vi "9_sub_Ntails.vi"(11 "Array":cluster{"PosX":i32, "PosY":i32}[](array[cluster])=[{"PosX"=0, "PosY"=0}, {"PosX"=0, "PosY"=1}, {"PosX"=0, "PosY"=2}, {"PosX"=0, "PosY"=3}, {"PosX"=0, "PosY"=3}, {"PosX"=1, "PosY"=4}, {"PosX"=2, "PosY"=4}, {"PosX"=3, "PosY"=4}, {"PosX"=3, "PosY"=4}, {"PosX"=4, "PosY"=3}, {"PosX"=4, "PosY"=2}, {"PosX"=4, "PosY"=2}, {"PosX"=4, "PosY"=2}, {"PosX"=4, "PosY"=2}, {"PosX"=3, "PosY"=3}, {"PosX"=3, "PosY"=4}, {"PosX"=3, "PosY"=4}, {"PosX"=3, "PosY"=4}, {"PosX"=3, "PosY"=4}, {"PosX"=2, "PosY"=3}, {"PosX"=2, "PosY"=2}, {"PosX"=2, "PosY"=1}, {"PosX"=2, "PosY"=1}, {"PosX"=2, "PosY"=1}]) -> (3 "Array 2":cluster{"PosX":i32, "PosY":i32}[](array[cluster]))   [LabVIEW 2021, in "2022.lvlib"]
uses:
  2022.lvlib
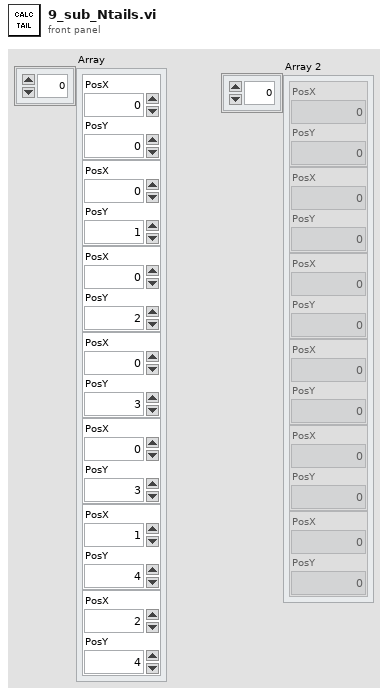
[diagram p1: front panel]
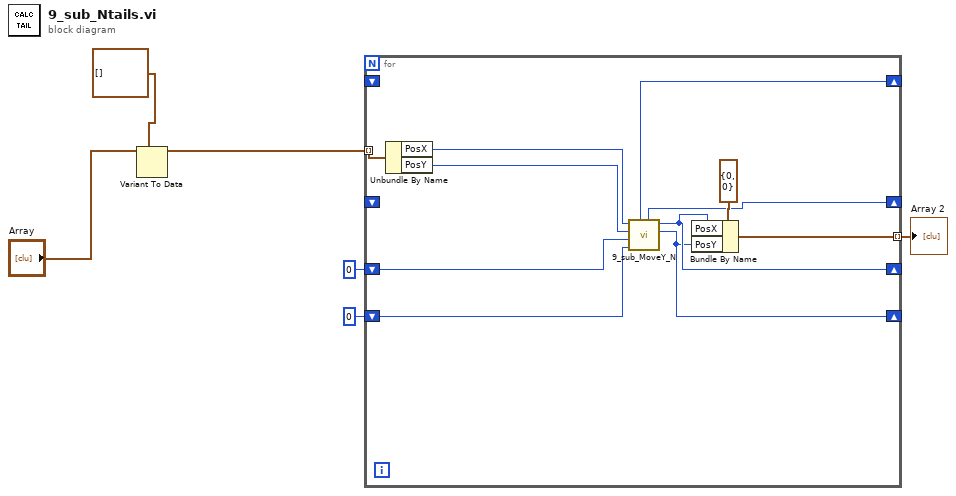
[diagram p0: block diagram]
diagram:
  n1 = Variant To Data(type=cluster{"PosX":i32, "PosY":i32}[] [], Variant="Array") -> (data=w5:cluster{"PosX":i32, "PosY":i32}[])  [unwired: 1 in, 1 out]
  n2 = for {
    shift-right: [w11] -> _
    shift-left: _ -> [_]
    shift-right: [w10] -> _
    shift-left: _ -> [_]
    shift-right: [w14] -> _
    shift-left: 0 ("T_x 2") -> [w17]
    shift-right: [w13] -> _
    shift-left: 0 ("T_y 2") -> [w16]
    tunnel: [w12] -> w4 mode=indexing
    tunnel: w5 -> [w9] mode=indexing
    n3 = Unbundle By Name(w9) -> ("PosX"=w8:i32, "PosY"=w7:i32)
    n4 = call "9_sub_MoveY_N.vi"("T_y"=w16, "T_x"=w17, "H_y"=w7, "H_x"=w8) -> ("T_y 2"=w13:i32, "T_x 2"=w14:i32, "H_y 2"=w10:i32, "H_x 2"=w11:i32)  [unwired: 4 in]
    n5 = Bundle By Name(cluster=cluster{"PosX":i32, "PosY":i32} {"PosX"=0, "PosY"=0} ("Tail"), "PosX"=w14, "PosY"=w13) -> (w12:cluster{"PosX":i32, "PosY":i32})
  }
  "Array 2" <- w4
